vi "Get Values.vi"(0 "image in":refnum<class "MSC Image.lvclass">, 5 "error in (no error)":errorcluster) -> (10 "picture":picture, 11 "imageData BGR":u32[][](array[numeric]), 14 "image out":refnum<class "MSC Image.lvclass">, 15 "imageData U8":u8[][](array[numeric]), 16 "imageData U16":u16[][](array[numeric]), 17 "imageData Single":sgl[][](array[numeric]), 18 "imageData Double":dbl[][](array[numeric]), 19 "error out":errorcluster)   [LabVIEW 2014, in "MSC Image.lvclass"]
doc: "Gets the array values of the image.\n\nUse the picture output for fast display rates."
uses:
  MSC Image.lvclass
  MSC Image.lvclass/MSC Image.ctl
  Dependencies/x86/MSC I Process32.dll
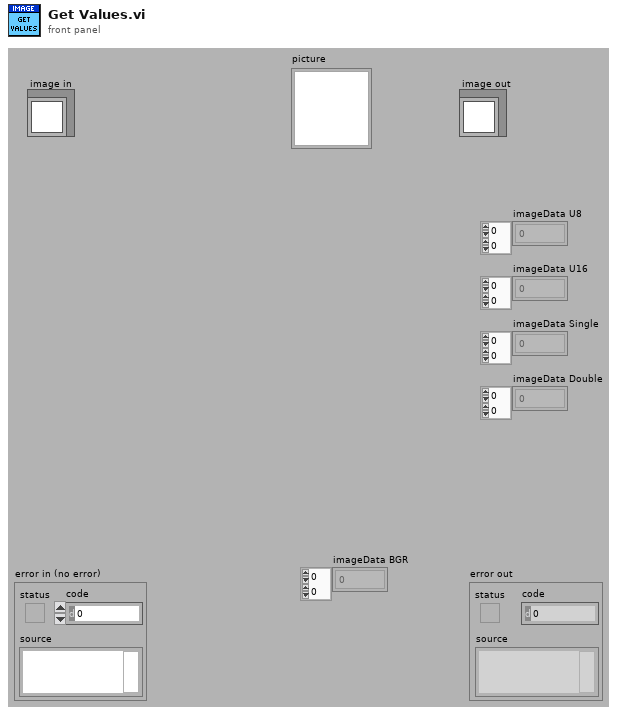
[diagram p1: front panel]
types:
  T1 = typedef "Image.ctl" = cluster{"Pointer":u64, "Size":T2, "Image Type":T3, "Time Stamp":timestamp, "Variant":variant}
  T2 = typedef "Size.ctl" = cluster{"Cols":i32, "Rows":i32}
  T3 = typedef "Image Type.ctl" = i32
  T4 = typedef "imagedata.ctl" = cluster{"image type":i32, "image depth":i32, "image":u8[], "mask":u8[], "colors":u32[], "Rectangle":cluster{"left":i16, "top":i16, "right":i16, "bottom":i16}}
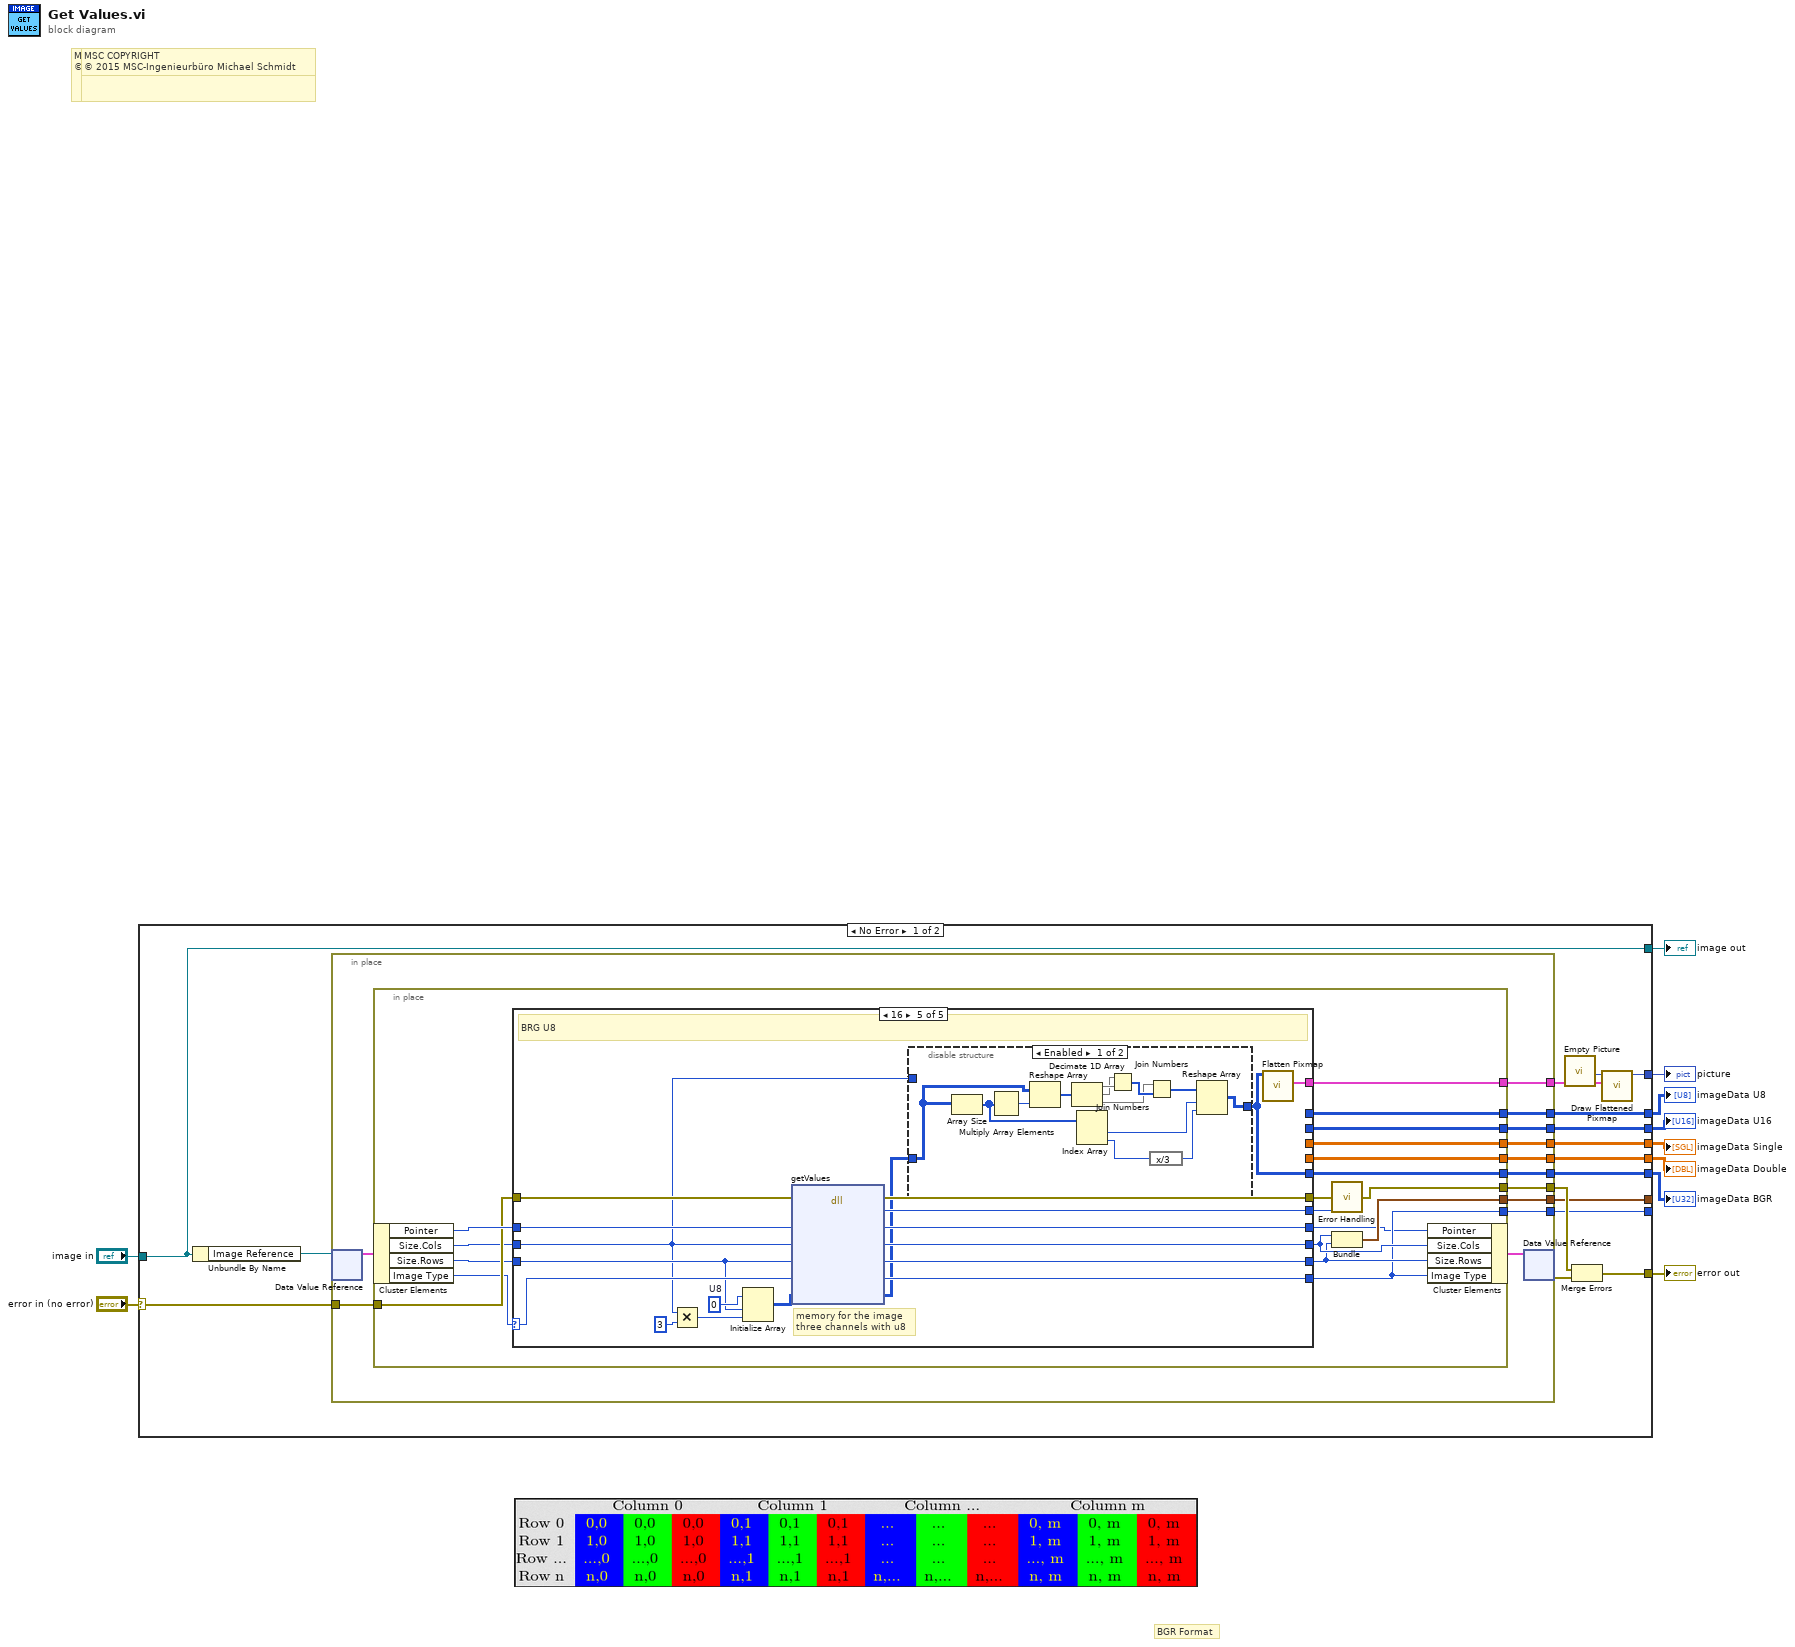
[diagram p0: block diagram]
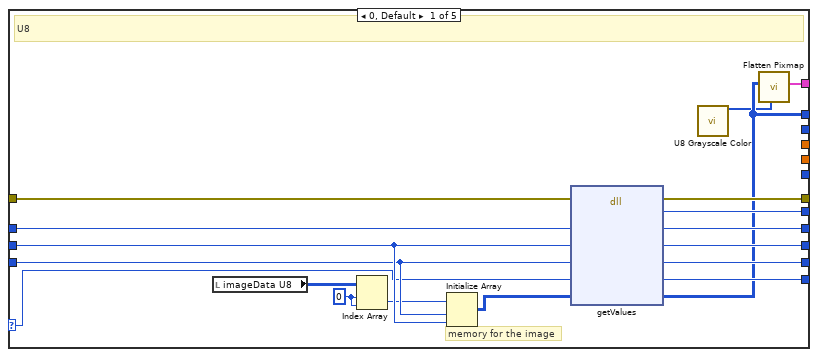
[diagram p2: hidden frame]
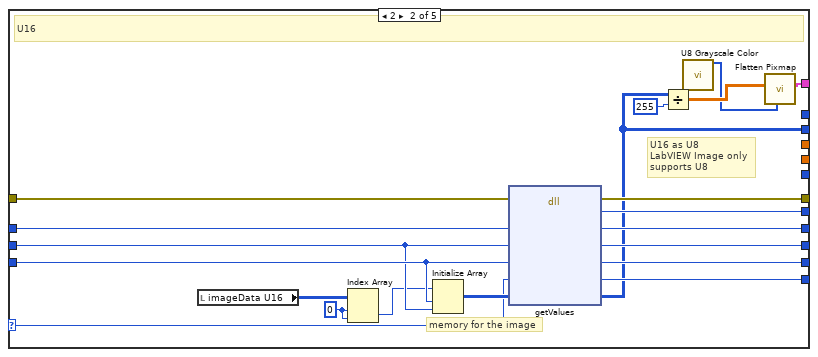
[diagram p3: hidden frame]
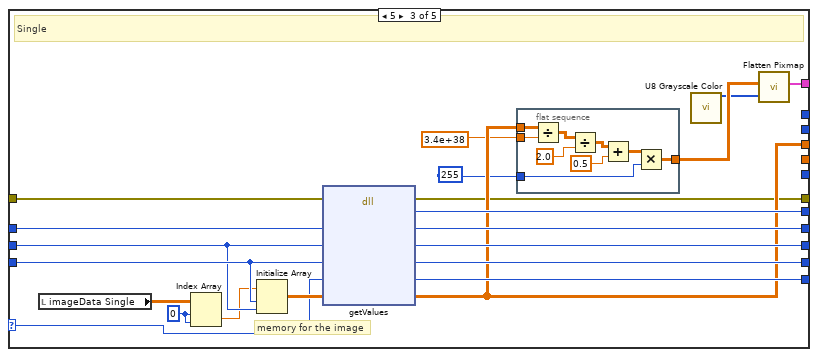
[diagram p4: hidden frame]
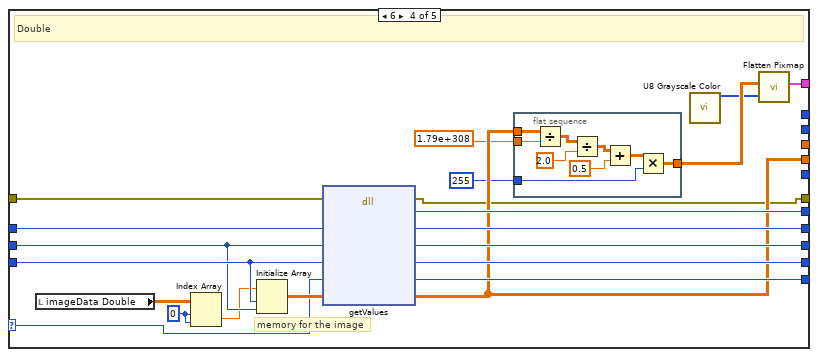
[diagram p5: hidden frame]
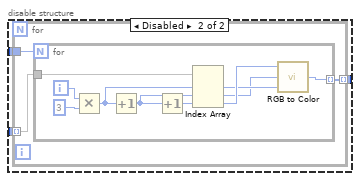
[diagram p6: hidden frame]
diagram:
  # "MSC COPYRIGHT\n© 2016 MSC-Ingenieurbüro Michael Schmidt"
  # "MSC COPYRIGHT\n© 2016 MSC-Ingenieurbüro Michael Schmidt"
  # "MSC COPYRIGHT\n© 2015 MSC-Ingenieurbüro Michael Schmidt"
  # "MSC COPYRIGHT\n© 2015 MSC-Ingenieurbüro Michael Schmidt"
  # "BGR Format"
  n1 = case shown="No Error" "error in (no error)" {
    selector: "error in (no error)" -> [w11 w204]
    tunnel: [w26 w204] -> w7
    tunnel: [w12 w203] -> w9
    tunnel: "image in" -> [w12 w203]
    tunnel: [w22 _] -> _
    tunnel: [w23 _] -> _
    tunnel: [w19 _] -> w1
    tunnel: [w18 _] -> w4
    tunnel: [w17 _] -> w6
    tunnel: [w16 _] -> w5
    tunnel: [w15 _] -> w2
    tunnel: [w14 _] -> w3
    frame No Error {
      n2 = Unbundle By Name(w12) -> ("Image Reference"=w13:refnum<data-value>)
      n3 = in-place {
        in-place-border: w11 -> [w36]
        in-place-border: [w35] -> w24
        in-place-border: [w34] -> w23
        in-place-border: [w33] -> w22
        in-place-border: [w32] -> w21
        in-place-border: [w31] -> w18
        in-place-border: [w30] -> w17
        in-place-border: [w29] -> w16
        in-place-border: [w28] -> w15
        in-place-border: [w27] -> w14
        n4 = in-place-dvr #1(w13) -> (w37:T1)  [unwired: 1 out]
        n5 = in-place {
          in-place-border: w36 -> [w54]
          in-place-border: [w53] -> w35
          in-place-border: [w48] -> w34
          in-place-border: [w47] -> w33
          in-place-border: [w46] -> w32
          in-place-border: [w44] -> w31
          in-place-border: [w43] -> w30
          in-place-border: [w41] -> w29
          in-place-border: [w42] -> w28
          in-place-border: [w40] -> w27
          n6 = in-place-cluster #2(w37) -> ("Pointer"=w57:u64, "Size.Cols"=w51:i32, "Size.Rows"=w52:i32, "Image Type"=w45:T3)
          n7 = case shown="16" w45 {
            selector: w45 -> [w59 w85 w107 w137 w165]
            tunnel: w57 -> [w75 w95 w116 w146 w173]
            tunnel: [w74 w94 w115 w145 w172] -> w39
            tunnel: [w73 w93 w97 w127 w171] -> w56
            tunnel: [w72 w92 w114 w144 w170] -> w55
            tunnel: w54 -> [w71 w91 w113 w143 w169]
            tunnel: w52 -> [w64 w90 w112 w142 w161]
            tunnel: w51 -> [w70 w89 w111 w141 w158]
            tunnel: [w68 w87 w109 w139 w167] -> w50
            tunnel: [w67 w86 w108 w138 w166] -> w49
            tunnel: [w66 w84 w106 w136 w164] -> w47
            tunnel: [w65 w82 w105 w135 w163] -> w46
            tunnel: [_ w80 _ _ _] -> w44
            tunnel: [_ _ _ _ w156] -> w43
            tunnel: [w60 _ _ _ _] -> w41
            tunnel: [_ _ _ w131 _] -> w42
            tunnel: [_ _ w101 _ _] -> w40
            frame 0, Default {
              w62 = 0 ("index (row)")
              # "memory for the image"
              # "U8"
              n8 = local read "imageData U8"() -> (w63:u8[][])
              n9 = Index Array(array=w63, index (row)=w62, index (col)=w62) -> (element=w61:u8)
              n10 = Initialize Array(w61, w64, w70) -> (w69:u8[][])
              n11 = dll-call lib="C:/Users/MSC/LabVIEW Projekte/LV 2014/MSC I-Process/user.lib/MSC-I Process/Dependencies/x86/MSC I Process*.dll" fn="getValues"(error in=w71, "pointer"=w75, "cols"=w70, "rows"=w64, "type"=w59, "imageData"=w69) -> (error out=w73:errorcluster, "error"=w72:i32, "pointer"=w74:u64, "cols"=w68:i32, "rows"=w67:i32, "type"=w66:i32, "imageData"=w60:u8[][])  [unwired: 2 in, 1 out]
              n12 = call "U8 Grayscale Color.vi"() -> ("Color Array"=w58:u32[])  [unwired: 15 in]
              n13 = call <vilib>:"Flatten Pixmap.vi"("colors"=w58, "8-bit pixmap"=w60) -> ("image data"=w65:T4)  [unwired: 9 in]
            }
            frame 2 {
              w78 = 0 ("index (row)")
              # "U16 as U8\nLabVIEW Image only\nsupports U8"
              # "memory for the image"
              # "U16"
              n14 = local read "imageData U16"() -> (w79:u16[][])
              n15 = Index Array(array=w79, index (row)=w78, index (col)=w78) -> (element=w77:u16)
              n16 = Initialize Array(w77, w90, w89) -> (w88:u16[][])
              n17 = dll-call lib="C:/Users/MSC/LabVIEW Projekte/LV 2014/MSC I-Process/user.lib/MSC-I Process/Dependencies/x86/MSC I Process*.dll" fn="getValues"(error in=w91, "pointer"=w95, "cols"=w89, "rows"=w90, "type"=w85, "imageData"=w88) -> (error out=w93:errorcluster, "error"=w92:i32, "pointer"=w94:u64, "cols"=w87:i32, "rows"=w86:i32, "type"=w84:i32, "imageData"=w80:u16[][])  [unwired: 2 in, 1 out]
              n18 = Divide(x=w80, y=u8 255) -> (x/y=w81:dbl[][])
              n19 = call "U8 Grayscale Color.vi"() -> ("Color Array"=w76:u32[])  [unwired: 15 in]
              n20 = call <vilib>:"Flatten Pixmap.vi"("colors"=w76, "8-bit pixmap"=w81) -> ("image data"=w82:T4)  [unwired: 9 in]
            }
            frame 5 {
              w102 = 0 ("index (row)")
              # "memory for the image"
              # "Single"
              n21 = local read "imageData Single"() -> (w104:sgl[][])
              n22 = Index Array(array=w104, index (row)=w102, index (col)=w102) -> (element=w103:sgl)
              n23 = Initialize Array(w103, w112, w111) -> (w110:sgl[][])
              n24 = dll-call lib="C:/Users/MSC/LabVIEW Projekte/LV 2014/MSC I-Process/user.lib/MSC-I Process/Dependencies/x86/MSC I Process*.dll" fn="getValues"(error in=w113, "pointer"=w116, "cols"=w111, "rows"=w112, "type"=w107, "imageData"=w110) -> (error out=w97:errorcluster, "error"=w114:i32, "pointer"=w115:u64, "cols"=w109:i32, "rows"=w108:i32, "type"=w106:i32, "imageData"=w101:sgl[][])  [unwired: 2 in, 1 out]
              n25 = flat-sequence {
                tunnel: [w121] -> w98
                tunnel: w101 -> [w120]
                tunnel: u8 255 ("y") -> [w118]
                tunnel: 3.4e+38 -> [w117]
                frame #0 {
                  n26 = Divide(x=w120, y=w117) -> (x/y=w125:dbl[][])
                  n27 = Divide(x=w125, y=2.0) -> (x/y=w124:dbl[][])
                  n28 = Add(x=w124, y=0.5) -> (x+y=w122:dbl[][])
                  n29 = Multiply(x=w122, y=w118) -> (x*y=w121:dbl[][])
                }
              }
              n30 = call "U8 Grayscale Color.vi"() -> ("Color Array"=w96:u32[])  [unwired: 15 in]
              n31 = call <vilib>:"Flatten Pixmap.vi"("colors"=w96, "8-bit pixmap"=w98) -> ("image data"=w105:T4)  [unwired: 9 in]
            }
            frame 6 {
              w132 = 0 ("index (row)")
              # "memory for the image"
              # "Double"
              n32 = local read "imageData Double"() -> (w134:dbl[][])
              n33 = Index Array(array=w134, index (row)=w132, index (col)=w132) -> (element=w133:dbl)
              n34 = Initialize Array(w133, w142, w141) -> (w140:dbl[][])
              n35 = dll-call lib="C:/Users/MSC/LabVIEW Projekte/LV 2014/MSC I-Process/user.lib/MSC-I Process/Dependencies/x86/MSC I Process*.dll" fn="getValues"(error in=w143, "pointer"=w146, "cols"=w141, "rows"=w142, "type"=w137, "imageData"=w140) -> (error out=w127:errorcluster, "error"=w144:i32, "pointer"=w145:u64, "cols"=w139:i32, "rows"=w138:i32, "type"=w136:i32, "imageData"=w131:dbl[][])  [unwired: 2 in, 1 out]
              n36 = flat-sequence {
                tunnel: [w151] -> w128
                tunnel: w131 -> [w150]
                tunnel: u8 255 ("y") -> [w148]
                tunnel: 1.79e+308 -> [w147]
                frame #0 {
                  n37 = Divide(x=w150, y=w147) -> (x/y=w155:dbl[][])
                  n38 = Divide(x=w155, y=2.0) -> (x/y=w154:dbl[][])
                  n39 = Add(x=w154, y=0.5) -> (x+y=w152:dbl[][])
                  n40 = Multiply(x=w152, y=w148) -> (x*y=w151:dbl[][])
                }
              }
              n41 = call "U8 Grayscale Color.vi"() -> ("Color Array"=w126:u32[])  [unwired: 15 in]
              n42 = call <vilib>:"Flatten Pixmap.vi"("colors"=w126, "8-bit pixmap"=w128) -> ("image data"=w135:T4)  [unwired: 9 in]
            }
            frame 16 {
              w162 = u8 0  # U8
              # "memory for the image\nthree channels with u8"
              # "BRG U8"
              n43 = Multiply(x=w158, y=3) -> (x*y=w159:i32)
              n44 = Initialize Array(w162, w161, w159) -> (w168:u8[][])
              n45 = dll-call lib="C:/Users/MSC/LabVIEW Projekte/LV 2014/MSC I-Process/user.lib/MSC-I Process/Dependencies/x86/MSC I Process*.dll" fn="getValues"(error in=w169, "pointer"=w173, "cols"=w158, "rows"=w161, "type"=w165, "imageData"=w168) -> (error out=w171:errorcluster, "error"=w170:i32, "pointer"=w172:u64, "cols"=w167:i32, "rows"=w166:i32, "type"=w164:i32, "imageData"=w157:u8[][])  [unwired: 2 in, 1 out]
              n46 = disable-structure shown="Enabled" {
                disable-tunnel: w158 -> [_ w189]
                disable-tunnel: w157 -> [w174 w188]
                disable-tunnel: [w175 w187] -> w156
                frame Enabled {
                  n47 = Array Size(array=w174) -> (size(s)=w179:i32[])
                  n48 = Multiply Array Elements(1:w179) -> (0:w182:i32)
                  n49 = Reshape Array(w174, w182) -> (w181:u8[])
                  n50 = Decimate 1D Array(w181) -> (w186:u8[], w185:u8[], w183:u8[])
                  n51 = Index Array(array=w179) -> (element #1=w178:i32, element #2=w177:i32)  [unwired: 2 in]
                  n52 = Join Numbers(hi=w185, lo=w186) -> ((hi.lo)=w184:u16[])
                  n53 = Join Numbers(hi=w183, lo=w184) -> ((hi.lo)=w180:u32[])
                  n54 = expression code="x/3"(w177) -> (w176:i32)
                  n55 = Reshape Array(w180, w178, w176) -> (w175:u32[][])
                }
                frame Disabled {
                  n56 = for {
                    tunnel: w188 -> [w192] mode=indexing
                    tunnel: [w191] -> w187 mode=indexing
                    tunnel: w189 -> [w190]
                    n57 = for {
                      N: w190 -> [_]
                      tunnel: w192 -> [w201]
                      tunnel: [w197] -> w191 mode=indexing
                      i -> [w196]
                      n58 = Multiply(x=w196, y=3) -> (x*y=w200:i32)
                      n59 = Increment(x=w200) -> (x+1=w199:i32)
                      n60 = Increment(x=w199) -> (x+1=w198:i32)
                      n61 = Index Array(array=w201, index #1=w200, index #2=w199, index #3=w198) -> (element #1=w194:u8, element #2=w193:u8, element #3=w195:u8)
                      n62 = call <vilib>:"RGB to Color.vi"("B"=w194, "G"=w193, "R"=w195) -> ("Color"=w197:u32)
                    }
                  }
                }
              }
              n63 = call <vilib>:"Flatten Pixmap.vi"("24-bit pixmap"=w156) -> ("image data"=w163:T4)  [unwired: 10 in]
            }
          }
          n64 = call "Error Handling.vi"("error in (no error)"=w56, "return type"=w55) -> ("error out"=w53:errorcluster)  [unwired: 12 in, 1 out]
          n65 = Bundle("cols"=w50, "rows"=w49) -> (w48:cluster{"cols":i32, "rows":i32})  [unwired: 1 in]
          n66 = in-place-cluster #2("Pointer"=w39, "Size.Cols"=w50, "Size.Rows"=w49, "Image Type"=w47) -> (w38:T1)
        }
        n67 = in-place-dvr #1(w38) -> (w25:errorcluster)  [unwired: 1 out]
      }
      n68 = call "Empty Picture"() -> ("empty picture"=w20:picture)
      n69 = Merge Errors(w24, w25) -> (w26:errorcluster)
      n70 = call <vilib>:"Draw Flattened Pixmap.vi"("image data"=w21, "picture"=w20) -> ("new picture"=w19:picture)  [unwired: 7 in]
    }
    frame Error {
    }
  }
  "error out" <- w7
  "image out" <- w9
  "imageData U16" <- w4
  "imageData U8" <- w5
  "imageData Double" <- w2
  "imageData Single" <- w3
  "picture" <- w1
  "imageData BGR" <- w6
